vi "reserve or unreserve tree entry.vi"(8 "error in (no error)":errorcluster, 9 "Item Ref in":T1 format="%.0x", 10 "Tag":string, 11 "TreeControl in":refnum<vi>) -> (0 "error out":errorcluster)   [LabVIEW 2016, in "FPGA Resource Manager.lvlib"]
uses:
  FPGA Resource Manager.lvlib
  <vilib>/NI Veristand/Custom Device API/Custom Device Item Ref.ctl
  tree reservation type.ctl
  <vilib>/NI VeriStand/Custom Device API/Custom Device API.lvlib
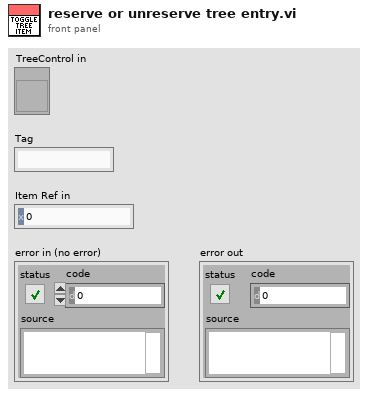
[diagram p1: front panel]
types:
  T1 = typedef "Custom Device API.lvlib/Custom Device Item Ref.ctl" = u64
  T2 = typedef "FPGA Resource Manager.lvlib/tree reservation type.ctl" = enum16{"none", "available", "reserved by this", "reserved by other", "incompatible", "parent"}
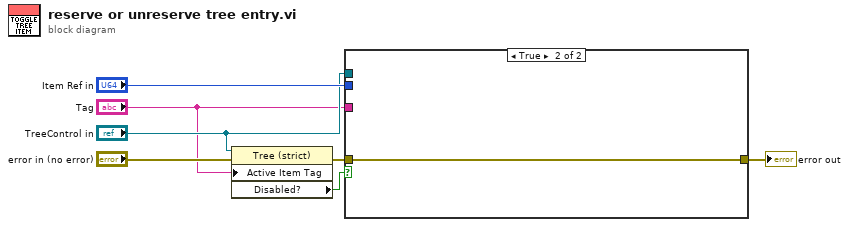
[diagram p0: block diagram]
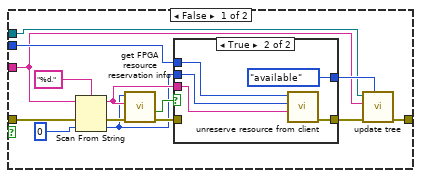
[diagram p2: hidden frame]
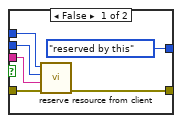
[diagram p3: hidden frame]
diagram:
  n1 = property class="Tree (strict)"(reference="TreeControl in", error in="error in (no error)", "Active Item Tag"="Tag") -> (error out=w3:errorcluster, "Disabled?"=w2:bool)  [unwired: 1 out]
  n2 = case shown="True" w2 {
    tunnel: [w20 w33] -> w7
    tunnel: w3 -> [w19 w33]
    tunnel: "Item Ref in" -> [w13 _]
    tunnel: "Tag" -> [w12 _]
    tunnel: "TreeControl in" -> [w8 _]
    frame False {
      n3 = Scan From String(format string="%d.", input string=w12, error in=w19, default 1=u64 0 ("default value 1")) -> (remaining string=w15:string, error out=w18:errorcluster, output 1=w14:u64)  [unwired: 1 in, 1 out]
      n4 = call "get FPGA resource reservation info.vi"("error in (no error)"=w18, "Name in Bitfile"=w15, "Item Ref in"=w14) -> ("error out"=w17:errorcluster, "found?"=w16:bool)  [unwired: 4 in, 3 out]
      n5 = case shown="True" w16 {
        tunnel: [w23 w32] -> w11
        tunnel: w13 -> [w26 w31]
        tunnel: w14 -> [w27 w30]
        tunnel: w15 -> [w25 w29]
        tunnel: w17 -> [w24 _]
        tunnel: [tree_reservation_type."reserved by this" ("status type") tree_reservation_type."available" ("status type")] -> w21
        frame False {
          n6 = call "reserve resource from client.vi"("error in (no error)"=w24, "Name in Bitfile"=w25, "Server Ref in"=w27, "Item Ref in"=w26) -> ("error out"=w23:errorcluster)  [unwired: 6 in, 1 out]
        }
        frame True {
          n7 = call "unreserve resource from client.vi"("Name in Bitfile"=w29, "Server Ref in"=w30, "Item Ref in"=w31) -> ("error out"=w32:errorcluster)  [unwired: 7 in, 1 out]
        }
      }
      n8 = call "update tree.vi"("status type"=w21, "error in (no error)"=w11, "tag"=w12, "TreeControl in"=w8) -> ("error out"=w20:errorcluster)  [unwired: 7 in]
    }
    frame True {
    }
  }
  "error out" <- w7
